vi "Check_Beam_Powers.vi"(3 "Mode":T6, 5 "Traverse line In":T3 {"Row Duration (mins)" format="%#.1f"; "Row No" min=0; "Trace Gas Concentration (%)" min=0.0 format="%#.2f"; "Emission Rate (l/min)" format="%#.2f"; "Tunnel Speed" format="%#.2f"; "Start X" format="%#.2f"; "Start Y" format="%#.2f"; "Start Z" format="%#.2f"; "End X" format="%#.2f"; "End Y" format="%#.2f"; "End Z" format="%#.2f"; "Averaging time (min)" min=0.0 format="%#.2f"}) -> (0 "Error Message":string, 1 "Status":T2, 2 "Traverse line Out":T3 {"Row Duration (mins)" format="%#.1f"; "Row No" min=0; "Trace Gas Concentration (%)" min=0.0 format="%#.2f"; "Emission Rate (l/min)" format="%#.2f"; "Tunnel Speed" format="%#.2f"; "Start X" format="%#.2f"; "Start Y" format="%#.2f"; "Start Z" format="%#.2f"; "End X" format="%#.2f"; "End Y" format="%#.2f"; "End Z" format="%#.2f"; "Averaging time (min)" min=0.0 format="%#.2f"})   [LabVIEW 2011]
uses:
  Gen Trav/Traverse_cluster.ctl
  Gen Trav/Spacing.ctl
  Controls/Multi_run_mode.ctl
  Controls/User_Specific_mode.ctl
  Gen Trav/Multi_Run_Status.ctl
  Controls/Beam_Type.ctl
  Gen Trav/Route mapping/Axis.ctl
  Controls/Save_Data.ctl
  Controls/Setup.ctl
  Globals/Meas_global.vi
  Globals/LDA_meas_global_1.vi
  Globals/LDA_meas_global_2.vi
panel:
  out "Light Power":dbl=8.10606551e-08 format="%^#_9e"
  in  "stop":bool
  out "Powers":dbl[](array[numeric]) format="%.4f"
  out "Beam Data":dbl[][](array[numeric]) format="%.4f"
  out "Beam Type":T1 items=["Green Unshifted", "Green Shifted", "Blue Unshifted", "Blue Shifted"]
  # "X                      Y                   Z          Datum Power"
  # "Green Unshifted\nGreen Shifted\nBlue Unshifted\nBlue Shifted"
  # "X           Y            Z"
  # "Start"
  # "End"
  # "X           Y            Z"
  # "Start"
  # "End"
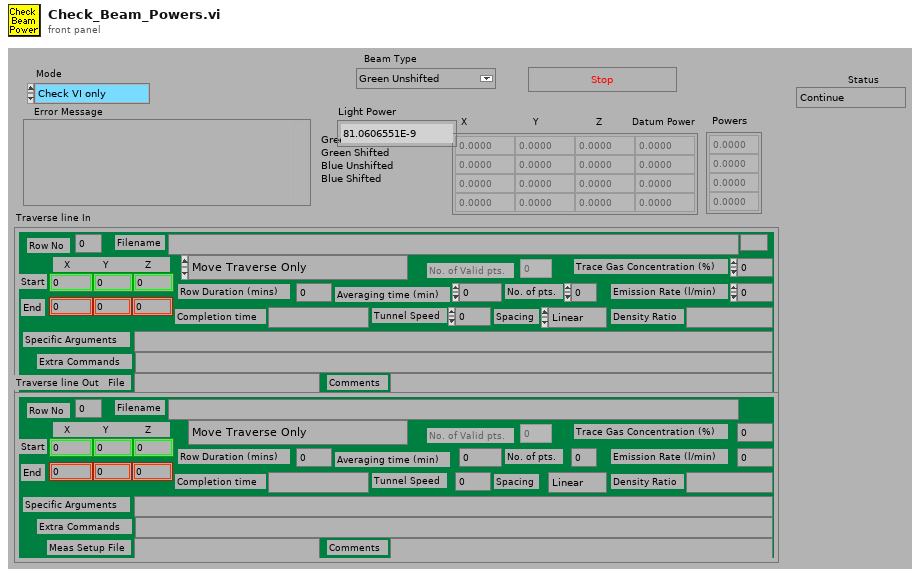
[diagram p1: front panel]
types:
  T1 = typedef "Beam_Type.ctl" = u16
  T2 = typedef "Multi_Run_Status.ctl" = enum16{"Continue", "Jump to Next Point", "Jump to Next Row", "Jump To Fall Back", "Terminate Run"}
  T3 = typedef "Traverse_cluster.ctl" = cluster{"Start X":dbl, "Start Y":dbl, "Start Z":dbl, "End X":dbl, "End Y":dbl, "End Z":dbl, "No. of pts.":i32, "Spacing":T4, "Filename":path, "Tunnel Speed":dbl, "Averaging time (min)":dbl, "Extra Commands":string, "Specific Arguments":string, "Emission Rate (l/min)":dbl, "Trace Gas Concentration (%)":dbl, "Density Ratio":string, "Comments":string, "Row No":i32, "Row Type Selector":T5, "Completion time":string, "Row Duration (mins)":dbl, "No. of Valid pts.":i32, "Meas Setup File":string}
  T4 = typedef "Spacing.ctl" = enum16{"Linear", "Log", "Gauss", "Specified", "N/A"}
  T5 = typedef "Multi_run_mode.ctl" = enum16{"Move Traverse Only", "Set Tunnel Speed Only", "Set Source Only", "Set Measurement Conditions", "Single Measurement", "Vertical Profile", "Lateral Profile", "Longitudinal Profile", "Explore Volume", "Multi-Axis Profile", "Auto Calibrate", "Meas Fast FID Bkgnd", "Check Beam Power", "Scanning Valve Measurement", "Run VI Named:", "Set ADAM Ch", "Wait (minutes)", "Send Message", "Synchronize With:", "Fall Back to this Row", "Turn Off Row Repeating", "Blank Row"}
  T6 = typedef "User_Specific_mode.ctl" = enum16{"Check VI only", "Run VI"}
  T7 = enum32{"Bad", "Idle", "Run top level", "Running"}
  T8 = enum16{"Load From Excel File", "Save to Excel File"}
  T9 = typedef "Axis.ctl" = enum16{"X Axis", "X Axis -ve", "Y Axis", "Y Axis -ve", "Z Axis", "Z Axis -ve"}
  T10 = typedef "Save_Data.ctl" = enum16{"Save No Data", "Save Data"}
  T11 = typedef "Setup.ctl" = enum16{"Run Program", "Show Setup", "Save Current Setup", "Setup Front Panel"}
  T12 = typedef "Status_Cluster.ctl" = cluster{"Status":T2, "Error Type":string, "Error Description":string}
  T13 = typedef "BSA_Type.ctl" = enum16{"57N11", "BSA F60"}
  T14 = typedef "BSA_info_Cluster.ctl" = cluster{"GPIB Address":string, "No of Check Bytes":i32, "Extra Info":string, "COLOUR":u32, "Wavelength (nm)":dbl}
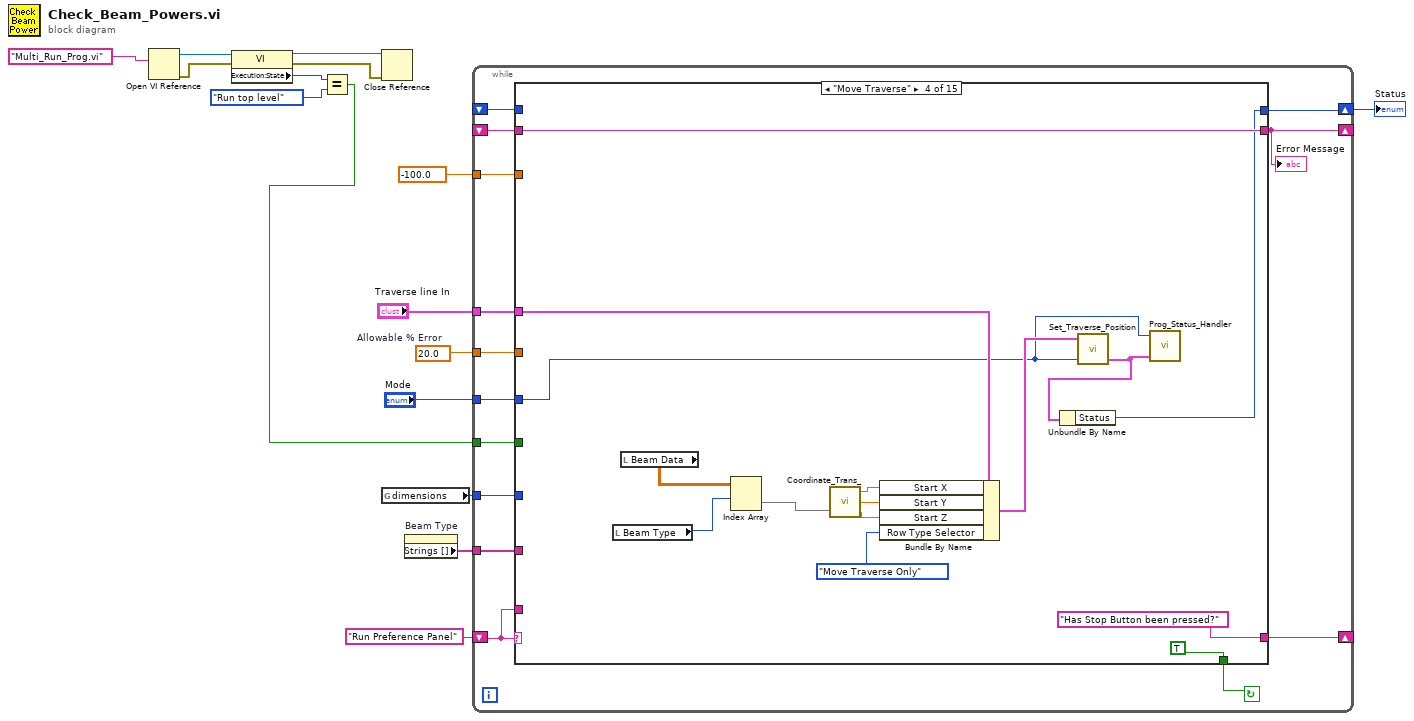
[diagram p0: block diagram]
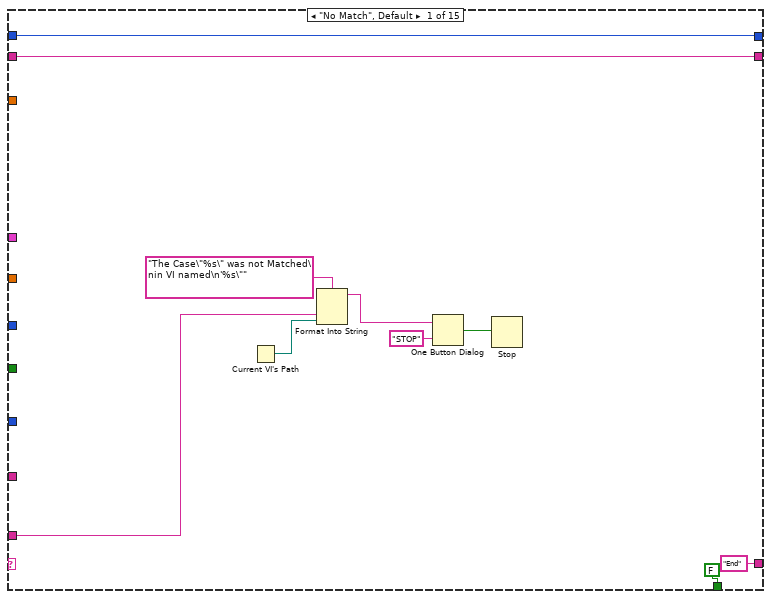
[diagram p2: hidden frame]
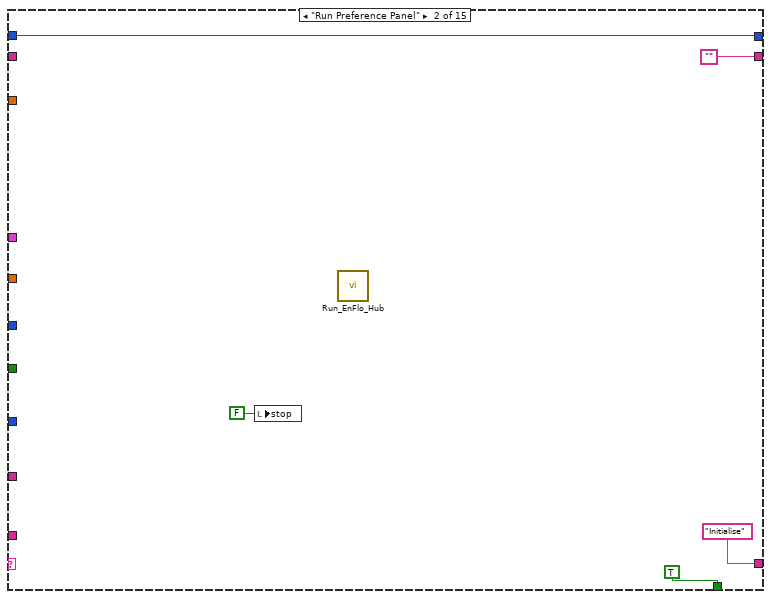
[diagram p3: hidden frame]
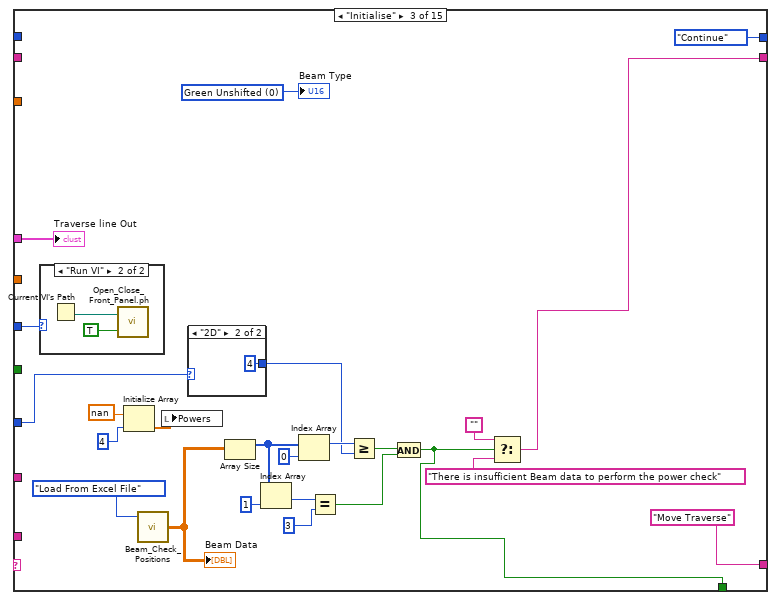
[diagram p4: hidden frame]
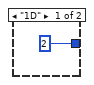
[diagram p5: hidden frame]
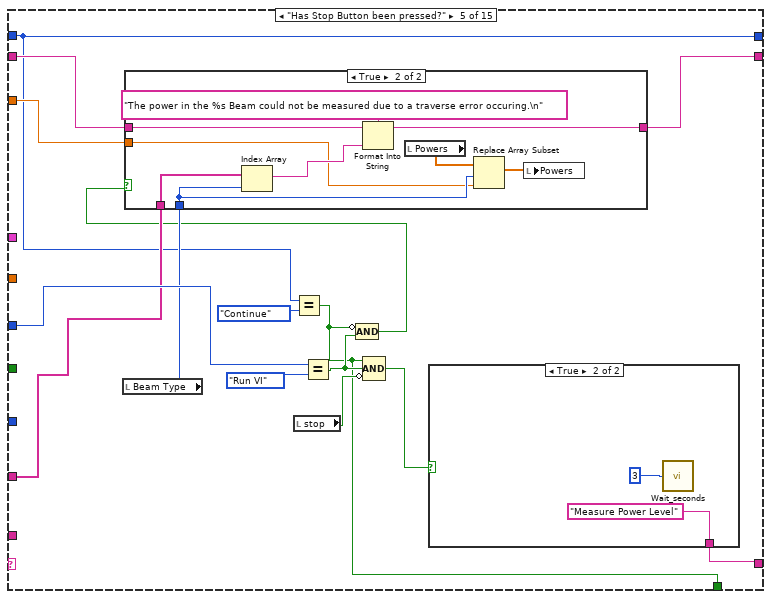
[diagram p7: hidden frame]
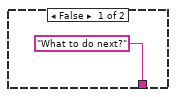
[diagram p9: hidden frame]
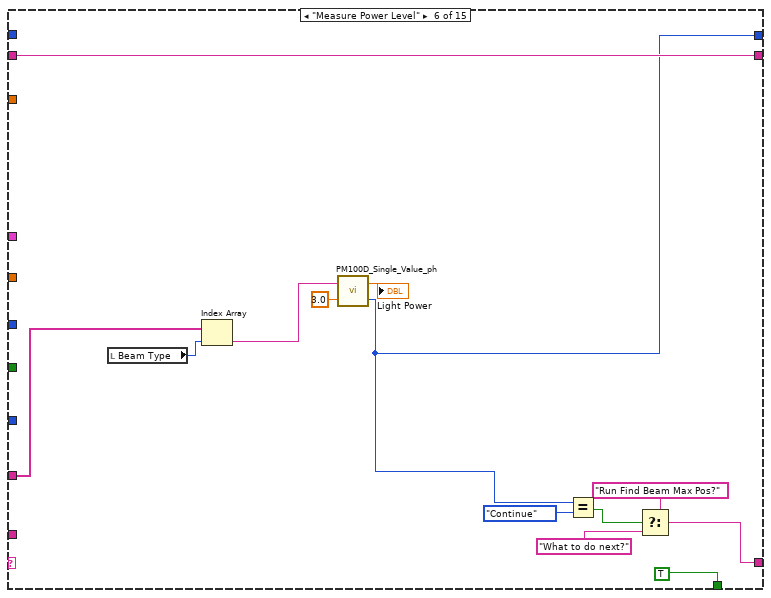
[diagram p10: hidden frame]
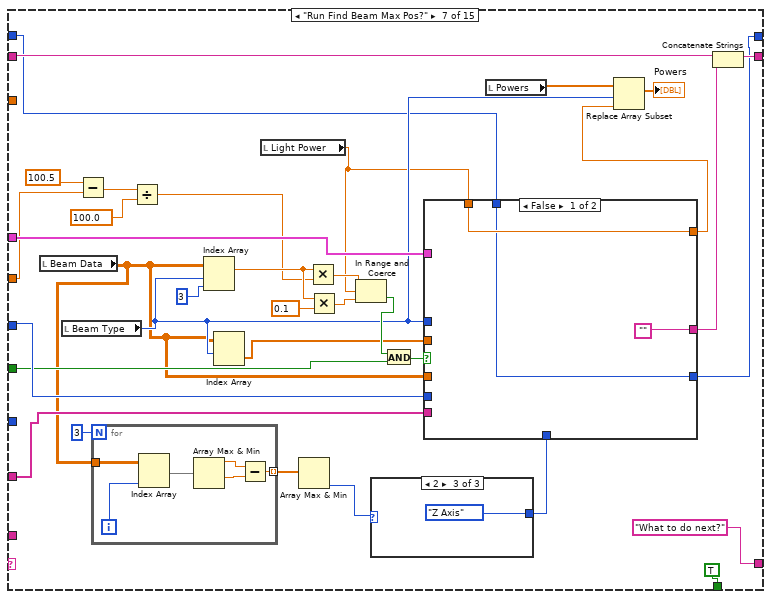
[diagram p11: hidden frame]
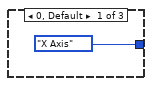
[diagram p12: hidden frame]
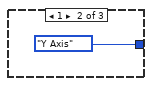
[diagram p13: hidden frame]
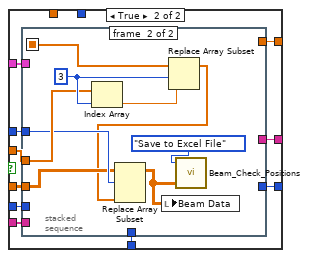
[diagram p14: hidden frame]
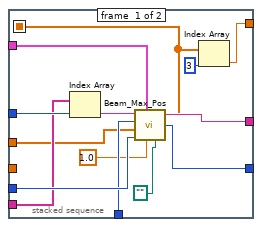
[diagram p15: hidden frame]
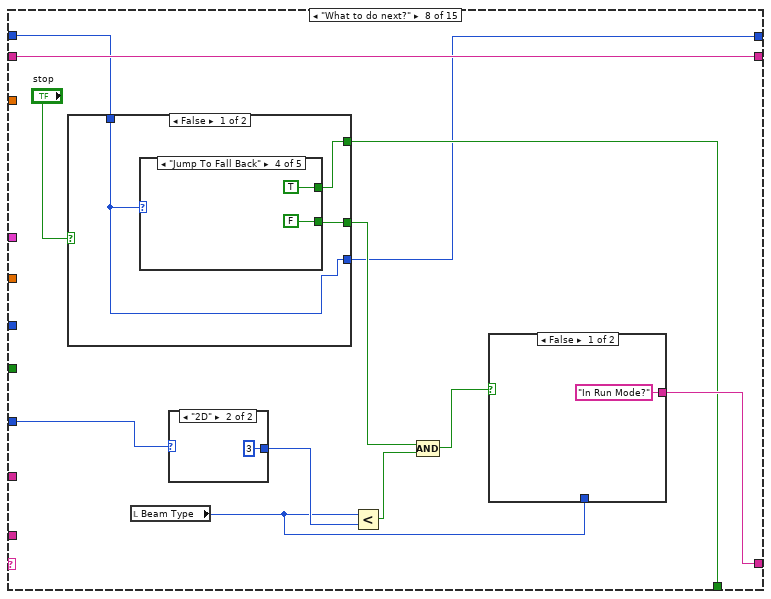
[diagram p16: hidden frame]
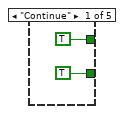
[diagram p17: hidden frame]
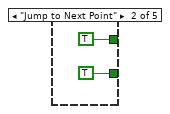
[diagram p18: hidden frame]
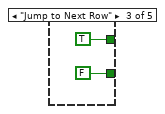
[diagram p19: hidden frame]
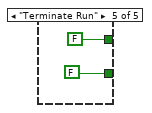
[diagram p20: hidden frame]
diagram:
  w12 = 20.0  # Allowable % Error
  n1 = Open VI Reference(vi path="Multi_Run_Prog.vi") -> (vi reference=w6:refnum<vi>, error out=w7:errorcluster)  [unwired: 1 in, 4 out]
  n2 = property class="VI"(reference=w6, error in=w7) -> (reference out=w8:refnum<vi>, error out=w9:errorcluster, "Execution:State"=w5:T7)
  n3 = Equal?(x=w5, y=T7."Run top level" ("Exec.State")) -> (x = y?=w3:bool)
  n4 = Close Reference(reference=w8, error in (no error)=w9) -> ()  [unwired: 1 out]
  n5 = global read "Meas_global.vi" "dimensions"() -> (w13:enum16{"1D", "2D"})
  n6 = property on="Beam Type" class="Ring (strict)"() -> ("Strings []"=w14:string[])  [unwired: 2 in, 2 out]
  n7 = while {
    tunnel: -100.0 ("Element Data") -> [w20]
    tunnel: w12 -> [w22]
    shift-left: _ -> [w24]
    shift-right: [w23] -> _
    tunnel: w13 -> [w25]
    tunnel: w14 -> [w28]
    tunnel: "Traverse line In" -> [w29]
    tunnel: "Mode" -> [w30]
    shift-left: "Run Preference Panel" -> [w21]
    shift-right: [w26] -> _
    tunnel: w3 -> [w19]
    shift-right: [w18] -> w1
    shift-left: _ -> [w17]
    stop <- w27 continue-if-true
    n8 = case shown="\"Move Traverse\"" w21 {
      tunnel: w29 -> [_ _ w67 w88 _ _ w162 _ _ _ _ _ _ w352 _]
      tunnel: w30 -> [_ _ w64 w83 w101 _ w161 _ w250 _ _ _ _ w356 w361]
      tunnel: w28 -> [_ _ _ _ w99 w119 w136 _ _ w267 _ _ _ _ _]
      tunnel: [FALSE ("Update Datum Powers?") TRUE ("Update Datum Powers?") w46 TRUE w90 TRUE TRUE w211 TRUE ("Update Datum Powers?") TRUE TRUE TRUE ("Update Datum Powers?") w322 w353 FALSE ("Update Datum Powers?")] -> w27
      tunnel: ["End" "Initialise" "Move Traverse" "Has Stop Button been pressed?" w100 w124 "What to do next?" w213 w245 "Log Beam Power Readings" w299 "Take datum velocity measurement?" "Move traverse to datum location" "Take a datum velocity measurement" "End"] -> w26
      tunnel: w25 -> [_ _ w63 _ _ _ _ w219 _ _ _ _ w324 _ _]
      tunnel: w24 -> [w32 _ _ w81 w97 w126 w148 w215 w249 w265 w294 w313 w326 w358 w364]
      tunnel: [w32 "" w47 w81 w98 w126 w147 w215 w249 w264 w294 "" w326 w358 w364] -> w23
      tunnel: w22 -> [_ _ _ _ _ _ w144 _ _ _ _ _ _ _ _]
      tunnel: w21 -> [w35 _ _ _ _ _ _ _ _ _ _ _ _ _ _]
      tunnel: w20 -> [_ _ _ _ w96 _ _ _ _ w262 _ _ _ _ _]
      tunnel: w19 -> [_ _ _ _ _ _ w137 _ _ _ _ _ w321 _ _]
      tunnel: [w31 w41 Multi_Run_Status."Continue" ("Status") w74 w89 w121 w131 w209 w243 w261 w297 w309 w319 w351 w360] -> w18
      tunnel: w17 -> [w31 w41 _ _ w89 _ w130 w210 w243 w261 w297 w309 w319 _ w359]
      frame "No Match", Default {
        n9 = Current VI's Path() -> (path=w36:path)
        n10 = Format Into String(format string="The Case\"%s\" was not Matched\nin VI named\n'%s\"" ("Format String"), w35, w36) -> (resulting string=w39:string)  [unwired: 2 in, 1 out]
        n11 = One Button Dialog(message=w39, button name ("OK")="STOP") -> (true=w37:bool)
        n12 = Stop(stop? (T)=w37) -> ()
      }
      frame "Run Preference Panel" {
        n13 = local write "stop"(FALSE ("stop")) -> ()
        n14 = call "Run_EnFlo_Hub.vi"() -> ()  [unwired: 8 out]
      }
      frame "Initialise" {
        w68 = T1 0 items=["Green Unshifted", "Green Shifted", "Blue Unshifted", "Blue Shifted"] ("Beam Type")
        n15 = case shown="\"Run VI\"" w64 {
          frame "Check VI only" {
          }
          frame "Run VI" {
            n16 = Current VI's Path() -> (path=w72:path)
            n17 = call "Open_Close_Front_Panel.ph.vi"("Front Panel Window:Open"=TRUE, "VI path"=w72) -> ()  [unwired: 2 out]
          }
        }
        n18 = Initialize Array(nan ("Numeric"), 4 ("Dimension Size")) -> (w50:dbl[])
        n19 = call "Beam_Check_Positions.vi"("Mode"=T8."Load From Excel File") -> ("Values Out"=w66:dbl[][])  [unwired: 1 in, 1 out]
        "Beam Data" <- w66
        n20 = local write "Powers"(w50) -> ()
        n21 = case shown="\"2D\"" w63 {
          tunnel: [2 4] -> w61
          frame "1D" {
          }
          frame "2D" {
          }
        }
        n22 = Array Size(array=w66) -> (size(s)=w57:i32[])
        n23 = Index Array(array=w57, index=1 ("Index")) -> (element=w56:i32)
        n24 = Index Array(array=w57, index=0 ("Index")) -> (element=w62:i32)
        n25 = Equal?(x=w56, y=3) -> (x = y?=w53:bool)
        n26 = Greater Or Equal?(x=w62, y=w61) -> (x >= y?=w54:bool)
        n27 = And(x=w54, y=w53) -> (x .and. y?=w46:bool)
        n28 = Select(t="", s=w46, f="There is insufficient Beam data to perform the power check") -> (s? t:f=w47:string)
        "Beam Type" <- w68
        "Traverse line Out" <- w67
      }
      frame "Move Traverse" {
        n29 = local read "Beam Type"() -> (w79:T1)
        n30 = local read "Beam Data"() -> (w80:dbl[][])
        n31 = Index Array(array=w80, index (row)=w79) -> (element=w75:dbl[])  [unwired: 1 in]
        n32 = call "Coordinate_Trans_.vi"("Input Position"=w75) -> ("X"=w78:dbl, "Y"=w77:dbl, "Z"=w76:dbl)  [unwired: 1 in]
        n33 = Bundle By Name(cluster=w88, "Start X"=w78, "Start Y"=w77, "Start Z"=w76, "Row Type Selector"=Multi_run_mode."Move Traverse Only") -> (w86:T3)
        n34 = call "Set_Traverse_Position.vi"("Simulate/Run"=w83, "Traverse line"=w86) -> ("Status Cluster"=w84:T12)  [unwired: 1 in, 2 out]
        n35 = Unbundle By Name(w84) -> ("Status"=w74:T2)
        n36 = call "Prog_Status_Handler.vi"("Status Cluster"=w84, "Simulate/Run"=w83) -> ()  [unwired: 2 out]
      }
      frame "Has Stop Button been pressed?" {
        n37 = local read "Beam Type"() -> (w95:T1)
        n38 = Equal?(x=w89, y=Multi_Run_Status."Continue" ("Status")) -> (x = y?=w90:bool)
        n39 = local read "stop"() -> (w94:bool)
        n40 = Equal?(x=w101, y=User_Specific_mode."Run VI" ("Mode")) -> (x = y?=w92:bool)
        n41 = Compound Arithmetic op=AND(invert w90, w92) -> (w91:bool)
        n42 = case shown="True" w91 {
          tunnel: w95 -> [_ w106]
          tunnel: w99 -> [_ w113]
          tunnel: w97 -> [w104 w110]
          tunnel: [w104 w109] -> w98
          tunnel: w96 -> [_ w105]
          frame False {
          }
          frame True {
            n43 = Index Array(array=w113, index=w106) -> (element=w112:string)
            n44 = Format Into String(format string="The power in the %s Beam could not be measured due to a traverse error occuring.\n" ("Format String"), initial string=w110, w112) -> (resulting string=w109:string)  [unwired: 1 in, 1 out]
            n45 = local read "Powers"() -> (w108:dbl[])
            n46 = Replace Array Subset(array=w108, new element=w105, index=w106) -> (w107:dbl[])
            n47 = local write "Powers"(w107) -> ()
          }
        }
        n48 = Compound Arithmetic op=AND(w90, w92, invert w94) -> (w93:bool)
        n49 = case shown="True" w93 {
          tunnel: ["What to do next?" "Measure Power Level"] -> w100
          frame False {
          }
          frame True {
            n50 = call "Wait_seconds.vi"("Seconds to wait"=u32 3) -> ()
          }
        }
      }
      frame "Measure Power Level" {
        n51 = local read "Beam Type"() -> (w120:T1)
        n52 = Index Array(array=w119, index=w120) -> (element=w118:string)
        n53 = call "PM100D_Single_Value_ph.vi"("Averaging Period (s)"=3.0, "Beam Name"=w118) -> ("Status"=w121:T2, "Light Power mW"=→"Light Power":dbl)
        n54 = Equal?(x=w121, y=Multi_Run_Status."Continue" ("Status")) -> (x = y?=w127:bool)
        n55 = Select(t="Run Find Beam Max Pos?", s=w127, f="What to do next?") -> (s? t:f=w124:string)
      }
      frame "Run Find Beam Max Pos?" {
        n56 = local read "Beam Data"() -> (w133:dbl[][])
        n57 = local read "Beam Type"() -> (w135:T1)
        n58 = Subtract(x=100.5, y=w144) -> (x-y=w143:dbl)
        n59 = for {
          N: 3 -> [_]
          tunnel: w133 -> [w171]
          tunnel: [w167] -> w159 mode=indexing
          i -> [w172]
          n60 = Index Array(array=w171, index (col)=w172) -> (element=w170:dbl[])  [unwired: 1 in]
          n61 = Array Max & Min(array=w170) -> (max value=w169:dbl, min value=w168:dbl)  [unwired: 2 out]
          n62 = Subtract(x=w169, y=w168) -> (x-y=w167:dbl)
        }
        n63 = Divide(x=w143, y=100.0) -> (x/y=w141:dbl)
        n64 = Index Array(array=w133, index (row)=w135, index (col)=3 ("Index")) -> (element=w155:dbl)
        n65 = Index Array(array=w133, index (row)=w135) -> (element=w134:dbl[])  [unwired: 1 in]
        n66 = local read "Light Power"() -> (w132:dbl)
        n67 = Array Max & Min(array=w159) -> (min index (indices)=w158:i32)  [unwired: 3 out]
        n68 = Multiply(x=w155, y=w141) -> (x*y=w153:dbl)
        n69 = Multiply(x=w155, y=0.1) -> (x*y=w152:dbl)
        n70 = In Range and Coerce(upper limit=w153, x=w132, lower limit=w152) -> (In Range?=w139:bool)  [unwired: 1 out]
        n71 = case shown="2" w158 {
          tunnel: [Axis."X Axis" ("Fixed Axis") Axis."Y Axis" ("Fixed Axis") Axis."Z Axis" ("Fixed Axis")] -> w157
          frame 0, Default {
          }
          frame 1 {
          }
          frame 2 {
          }
        }
        n72 = And(x=w139, y=w137) -> (x .and. y?=w138:bool)
        n73 = case shown="False" w138 {
          tunnel: w135 -> [_ w180]
          tunnel: w162 -> [_ w185]
          tunnel: w161 -> [_ w184]
          tunnel: w157 -> [_ w183]
          tunnel: [w175 w182] -> w149
          tunnel: w132 -> [w175 _]
          tunnel: ["" w181] -> w146
          tunnel: w136 -> [_ w179]
          tunnel: w134 -> [_ w178]
          tunnel: w133 -> [_ w177]
          tunnel: [w173 w176] -> w131
          tunnel: w130 -> [w173 _]
          frame False {
          }
          frame True {
            n74 = stacked-sequence {
              seq-local: [w188 _] -> [_ w206]
              tunnel: w185 -> [w199 _]
              tunnel: w184 -> [w198 _]
              tunnel: w183 -> [w197 _]
              tunnel: [w195 _] -> w182
              tunnel: [w194 _] -> w181
              tunnel: w180 -> [w192 w204]
              tunnel: w179 -> [w191 _]
              tunnel: w178 -> [w189 w205]
              tunnel: w177 -> [_ w203]
              tunnel: [w186 _] -> w176
              frame #0 {
                n75 = Index Array(array=w191, index=w192) -> (element=w190:string)
                n76 = call "Beam_Max_Pos.vi"("Picture Log"=path "", "Search Step (mm)"=1.0, "Mode"=w198, "Starting Position"=w189, "Traverse line In"=w199, "Fixed Axis"=w197, "Beam Name"=w190) -> ("Status"=w186:T2, "Beam maxima"=w188:dbl[], "Message"=w194:string)  [unwired: 1 out]
                n77 = Index Array(array=w188, index=3 ("Index")) -> (element=w195:dbl)
              }
              frame #1 {
                w207 = 3 ("index")
                n78 = Index Array(array=w205, index=w207) -> (element=w208:dbl)
                n79 = Replace Array Subset(array=w206, new element=w208, index=w207) -> (w200:dbl[])
                n80 = Replace Array Subset(array=w203, new element=w200, index (row)=w204) -> (w202:dbl[][])  [unwired: 1 in]
                n81 = local write "Beam Data"(w202) -> ()
                n82 = call "Beam_Check_Positions.vi"("Values"=w202, "Mode"=T8."Save to Excel File") -> ()  [unwired: 2 out]
              }
            }
          }
        }
        n83 = local read "Powers"() -> (w151:dbl[])
        n84 = Replace Array Subset(array=w151, new element=w149, index=w135) -> (→"Powers":dbl[])
        n85 = Concatenate Strings(w148, w146) -> (w147:string)
      }
      frame "What to do next?" {
        n86 = case shown="False" "stop" {
          tunnel: [w223 FALSE] -> w212
          tunnel: [w222 FALSE] -> w211
          tunnel: w210 -> [w221 _]
          tunnel: [w221 Multi_Run_Status."Terminate Run" ("Status")] -> w209
          frame False {
            n87 = case shown="\"Jump To Fall Back\"" w221 {
              tunnel: [TRUE TRUE FALSE FALSE FALSE] -> w223
              tunnel: [TRUE TRUE TRUE TRUE FALSE] -> w222
              frame "Continue" {
              }
              frame "Jump to Next Point" {
              }
              frame "Jump to Next Row" {
              }
              frame "Jump To Fall Back" {
              }
              frame "Terminate Run" {
              }
            }
          }
          frame True {
          }
        }
        n88 = local read "Beam Type"() -> (w216:T1)
        n89 = case shown="\"2D\"" w219 {
          tunnel: [1 3] -> w220
          frame "1D" {
          }
          frame "2D" {
          }
        }
        n90 = Less?(x=w216, y=w220) -> (x < y?=w218:bool)
        n91 = Compound Arithmetic op=AND(w212, w218) -> (w217:bool)
        n92 = case shown="False" w217 {
          tunnel: w216 -> [_ w240]
          tunnel: ["In Run Mode?" "Move Traverse"] -> w213
          frame False {
          }
          frame True {
            n93 = Increment(x=w240) -> (x+1=w239:T1)
            n94 = local write "Beam Type"(w239) -> ()
          }
        }
      }
      frame "In Run Mode?" {
        n95 = Equal?(x=w250, y=User_Specific_mode."Run VI" ("Mode")) -> (x = y?=w247:bool)
        n96 = Select(t="Are Powers Acceptable?", s=w247, f="Move traverse to datum location") -> (s? t:f=w245:string)
      }
      frame "Are Powers Acceptable?" {
        n97 = global read "LDA_meas_global_1.vi" "Min Green Unshifted Power mW"() -> (w253:i32)
        n98 = global read "LDA_meas_global_1.vi" "Min Blue Unshifted Power mW"() -> (w255:i32)
        n99 = global read "LDA_meas_global_1.vi" "Min Green Shifted Power mW"() -> (w254:i32)
        n100 = global read "LDA_meas_global_1.vi" "Min Blue Shifted Power mW"() -> (w256:i32)
        n101 = local read "Powers"() -> (w268:dbl[])
        n102 = Build Array(w253, w254, w255, w256) -> (w257:i32[])
        n103 = To Double Precision Float(number=w257) -> (double precision float=w252:dbl[])
        n104 = for {
          tunnel: w268 -> [w275] mode=indexing
          tunnel: w252 -> [w274] mode=indexing
          shift-right: [w284] -> w259
          shift-left: "" -> [w286]
          tunnel: w267 -> [w285] mode=indexing
          tunnel: w262 -> [w279]
          n105 = Subtract(x=w275, y=w274) -> (x-y=w280:dbl)
          n106 = Divide(x=w280, y=w274) -> (x/y=w282:dbl)
          n107 = Not Equal?(x=w279, y=w275) -> (x != y?=w276:bool)
          n108 = Absolute Value(x=w282) -> (abs(x)=w281:dbl)
          n109 = Multiply(x=w281, y=100.0) -> ()  [unwired: 1 out]
          n110 = Less Than 0?(x=w280) -> (x < 0?=w277:bool)
          n111 = Compound Arithmetic op=AND(w276, w277) -> (w278:bool)
          n112 = case shown="True" w278 {
            tunnel: w286 -> [w287 w292]
            tunnel: w285 -> [_ w293]
            tunnel: [w287 w291] -> w284
            tunnel: w275 -> [_ w289]
            tunnel: w274 -> [_ w288]
            frame False {
            }
            frame True {
              n113 = Format Into String(format string="The %s laser beam power is %.1f mW. It lowest acceptable power has been set to %.1f mW. \\n" ("Format String"), initial string=w292, w293, w289, w288) -> (resulting string=w291:string)  [unwired: 1 in, 1 out]
            }
          }
        }
        n114 = Empty String/Path?(string/path=w259) -> (empty?=w260:bool)
        n115 = case shown="False" w260 {
          tunnel: w259 -> [w271 w273]
          tunnel: [w270 w273] -> w258
          frame False {
            n116 = Concatenate Strings(w271, "Please come and check the system As Soon As Possible!\nThe probe may have collided with something or the optical fibres could be getting damaged due to poor launch efficiency! £18,000 TO REPAIR!!\nThe Multi Run will continue." ("Substring")) -> (w270:string)
          }
          frame True {
          }
        }
        n117 = Concatenate Strings(w265, w258) -> (w264:string)
      }
      frame "Log Beam Power Readings" {
        n118 = local read "Beam Data"() -> (w302:dbl[][])
        n119 = local read "Powers"() -> (w301:dbl[])
        n120 = for {
          tunnel: w302 -> [w308] mode=indexing
          tunnel: w301 -> [w305] mode=indexing
          tunnel: [w304] -> w300 mode=indexing
          n121 = Array Subset(array=w308, length=3 ("Array Length")) -> (w306:dbl[])  [unwired: 1 in]
          n122 = Build Array (concatenate)(w306, w305) -> (w304:dbl[])
        }
        n123 = Empty String/Path?(string/path=w294) -> (empty?=w295:bool)
        n124 = call "Log_beam_power.vi"("Message"=w294, "Beam Data"=w300) -> ()  [unwired: 4 out]
        n125 = Select(t="Take datum velocity measurement?", s=w295, f="Send Error Email") -> (s? t:f=w299:string)
      }
      frame "Send Error Email" {
        w317 = FALSE  # Dialog Box (T)
        n126 = Bundle By Name(cluster=errorcluster {"status"=FALSE, "code"=0, "source"=""} ("error in (no error)"), "source"=w313, "status"=TRUE ("Bundle Element")) -> (w315:errorcluster)
        n127 = call "EnFlo_Error_Handler.vi"("error in (no error)"=w315, "Error Type"="Beam Power", "Dialog Box (T)"=w317) -> ()  [unwired: 3 out]
      }
      frame "Take datum velocity measurement?" {
        n128 = global read "LDA_meas_global_1.vi" "BSA Type"() -> (w320:T13)
        n129 = case shown="\"57N11\"" w320 {
          tunnel: w324 -> [w329 _]
          tunnel: [w328 TRUE] -> w323
          tunnel: w321 -> [w327 _]
          frame "57N11" {
            n130 = stacked-sequence {
              tunnel: w329 -> [_ w342]
              tunnel: [_ w338] -> w328
              tunnel: w327 -> [w330 _]
              frame #0 {
                n131 = case shown="True" w330 {
                  frame False {
                  }
                  frame True {
                    n132 = stacked-sequence {
                      frame #0 {
                        n133 = global read "LDA_meas_global_2.vi" "BSA2 info"() -> (w331:T14)
                        n134 = global read "LDA_meas_global_1.vi" "BSA1 info"() -> (w336:T14)
                        n135 = Unbundle By Name(w331) -> ("GPIB Address"=w332:string)
                        n136 = Unbundle By Name(w336) -> ("GPIB Address"=w335:string)
                        n137 = call "Set_BSA_voltage_On_Off.vi"("GPIB address"=w332, "High Voltage"=TRUE) -> ()  [unwired: 1 in, 5 out]
                        n138 = call "Set_BSA_voltage_On_Off.vi"("GPIB address"=w335, "High Voltage"=TRUE) -> ()  [unwired: 1 in, 5 out]
                      }
                      frame #1 {
                        n139 = call "Wait_seconds.vi"("Seconds to wait"=u32 5) -> ()
                      }
                    }
                  }
                }
              }
              frame #1 {
                w339 = 7.0 ("y")
                n140 = call "LDA_data_rate.vi"() -> ("Data rate (Hz) BSA1"=w343:dbl, "Data rate (Hz) BSA2"=w340:dbl)  [unwired: 1 out]
                n141 = Greater?(x=w343, y=w339) -> (0:w341:bool)
                n142 = case shown="\"1D\"" w342 {
                  tunnel: w341 -> [w344 w348]
                  tunnel: w340 -> [_ w347]
                  tunnel: w339 -> [_ w346]
                  tunnel: [w344 w345] -> w338
                  frame "1D" {
                  }
                  frame "2D" {
                    n143 = Greater?(x=w347, y=w346) -> (0:w349:bool)
                    n144 = And(x=w348, y=w349) -> (x .and. y?=w345:bool)
                  }
                }
              }
            }
          }
          frame "BSA F60" {
          }
        }
        n145 = And(x=w323, y=w321) -> (x .and. y?=w322:bool)
      }
      frame "Move traverse to datum location" {
        n146 = call "Set_Traverse_Position.vi"("Simulate/Run"=w356, "Traverse line"=w352) -> ("Status Cluster"=w355:T12)  [unwired: 1 in, 2 out]
        n147 = Unbundle By Name(w355) -> ("Status"=w351:T2)
        n148 = Equal?(x=Multi_Run_Status."Continue" ("Status"), y=w351) -> (x = y?=w353:bool)
      }
      frame "Take a datum velocity measurement" {
        n149 = case shown="\"Run VI\"" w361 {
          tunnel: [w365 w366] -> w360
          tunnel: w359 -> [w365 _]
          frame "Check VI only" {
          }
          frame "Run VI" {
            n150 = flat-sequence {
              tunnel: [w371] -> w368
              tunnel: [w370] -> w367
              tunnel: [w369] -> w366
              tunnel: w368 -> [w380]
              tunnel: w367 -> [w379]
              frame #0 {
                w373 = 1.0  # Averaging time (min)
                w376 = FALSE  # Acquisition Interlock
                w377 = FALSE  # Open Front Panel
                w378 = FALSE  # Remote control
                n151 = call "Create_Error_log_folders.vi"("Log Filename"="LDA_Datum_Vel.xls" ("Input Element")) -> ("Server copy Location"=w370:path, "Local Log File"=w371:path)  [unwired: 2 in, 1 out]
                n152 = call "Code_to_run.vi"("Open Front Panel"=w377, "Acquisition Interlock"=w376, "setup"=Setup."Run Program", "Remote control"=w378, "File"=Save_Data."Save Data", "Results Filename"=w371, "Averaging time (min)"=w373) -> ("Status"=w369:T2)  [unwired: 4 in, 4 out]
              }
              frame #1 {
                n153 = call "Updated_File_Copy.vi"("Target Path"=w379, "Source Path"=w380) -> ()  [unwired: 2 out]
              }
            }
          }
        }
      }
    }
    "Error Message" <- w23
  }
  "Status" <- w1
